vi "SE FP hindbrain SENSE.vi"(2 "GPS":cluster{"X pos":i32, "Y pos":i32, "Heading":dbl}, 3 "error in":errorcluster, 4 "Analog Input Values":dbl[](array[numeric]), 5 "IR Sensors":T2(array[cluster])) -> (0 "error out":errorcluster, 1 "Boat Status":T1)   [LabVIEW 2014]
doc: "This vi calculate the distance from the boat edge to the detected object. If no object is detected the value is 0. It also determines of the boat is out of power...if so it will stop the boat."
panel:
  out "RIO BAT":dbl
  out "MOT BAT":dbl
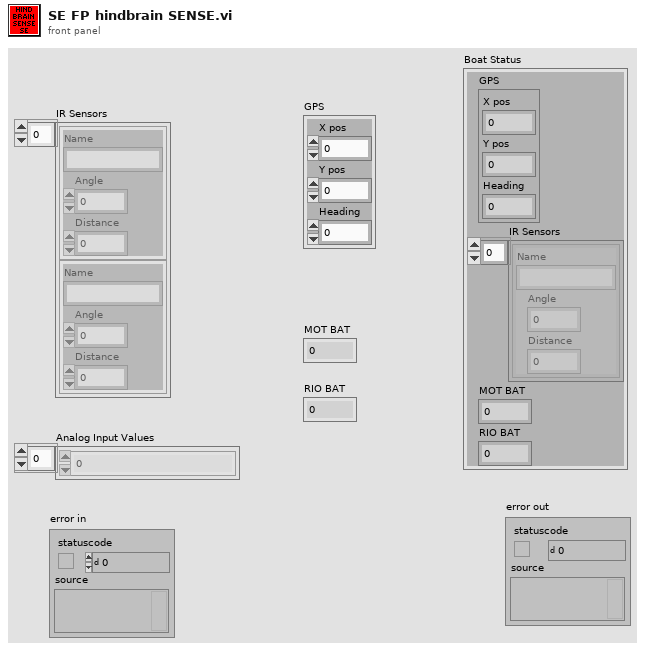
[diagram p1: front panel]
types:
  T1 = cluster{"GPS":cluster{"X pos":i32, "Y pos":i32, "Heading":dbl}, "IR Sensors":cluster{"Name":string, "Angle":dbl, "Distance":dbl}[], "MOT BAT":dbl, "RIO BAT":dbl}
  T2 = cluster{"Name":string, "Angle":dbl, "Distance":dbl}[]
  T3 = cluster{"Name":string, "Angle":dbl, "Distance":dbl}
  T4 = cluster{"GPS":cluster{"X pos":i32, "Y pos":i32, "Heading":dbl}, cluster{"Name":string, "Angle":dbl, "Distance":dbl}[], "MOT BAT":dbl, "RIO BAT":dbl}
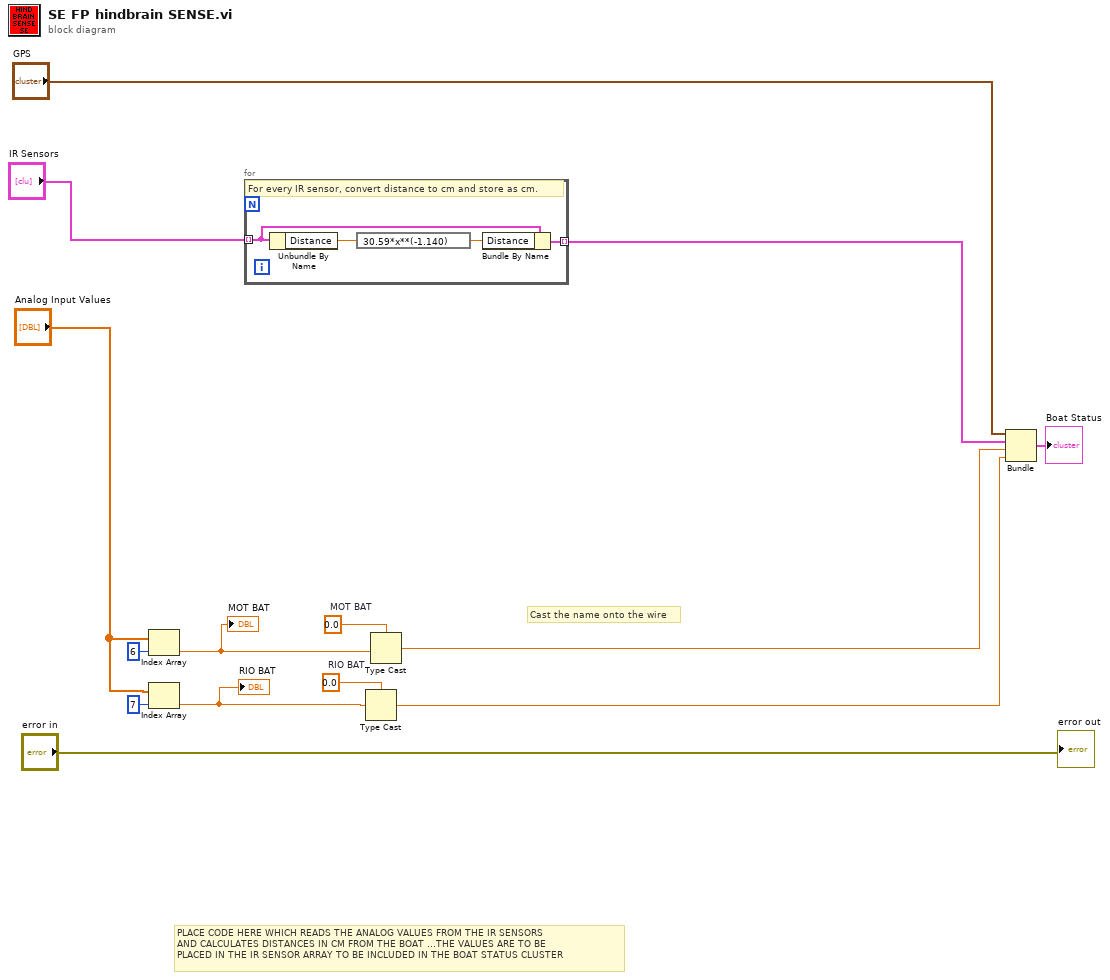
[diagram p0: block diagram]
diagram:
  w6 = 0.0  # RIO BAT
  w11 = 0.0  # MOT BAT
  # "PLACE CODE HERE WHICH READS THE ANALOG VALUES FROM THE IR SENSORS \nAND CALCULATES DISTANCES IN CM FROM THE BOAT ...THE VALUES ARE TO BE \nPLACED IN THE IR SENSOR ARRAY TO BE INCLUDED IN THE BOAT STATUS CLUSTER"
  # "Cast the name onto the wire"
  n1 = Index Array(array="Analog Input Values", index=6) -> (element=w10:dbl)
  "MOT BAT" <- w10
  n2 = Index Array(array="Analog Input Values", index=7) -> (element=w5:dbl)
  "RIO BAT" <- w5
  n3 = for {
    tunnel: "IR Sensors" -> [w16] mode=indexing
    tunnel: [w15] -> w1 mode=indexing
    # "For every IR sensor, convert distance to cm and store as cm."
    n4 = Unbundle By Name(w16) -> ("Distance"=w18:dbl)
    n5 = expression code="30.59*x**(-1.140)"(w18) -> (w17:dbl)
    n6 = Bundle By Name(cluster=w16, "Distance"=w17) -> (w15:T3)
  }
  n7 = Type Cast(type=w6, x=w5) -> (*(type *) &x=w4:dbl)
  n8 = Type Cast(type=w11, x=w10) -> (*(type *) &x=w9:dbl)
  n9 = Bundle("GPS"="GPS", w1, "MOT BAT"=w9, "RIO BAT"=w4) -> (→"Boat Status":T4)  [unwired: 1 in]
  "error out" <- "error in"
